vi "LCA Get Axis Handle.vi"(8 "error in (no error)":errorcluster caption="Fehler (Eingang, kein Fehler)", 10 "Axis Index":u8, 11 "Axis System Handle":i64) -> (0 "error out":errorcluster caption="Fehler (Ausgang)", 3 "AxisHandle":i64)   [LabVIEW 2021, in "labbCAN_MotionControl_API.lvlib"]
doc: "LCA_Func dev_hdl __stdcall LCA_GetAxisHandle(dev_hdl hAxisSystem,\n unsigned char AxisId);"
uses:
  labbCAN_MotionControl_API.lvlib
  labbCAN_MotionControl_API.dll
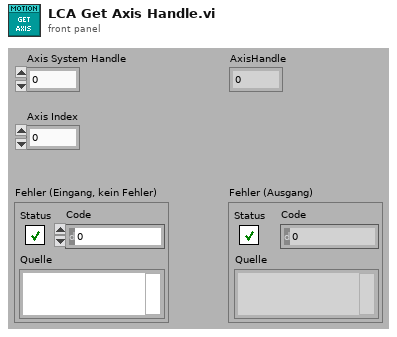
[diagram p1: front panel]
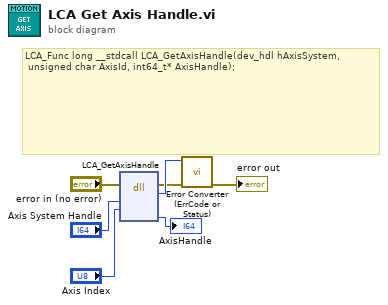
[diagram p0: block diagram]
diagram:
  # "LCA_Func long __stdcall LCA_GetAxisHandle(dev_hdl hAxisSystem,\n\tunsigned char AxisId, int64_t* AxisHandle);"
  n1 = dll-call lib="C:/Users/olaja/AppData/Local/CETONI_SDK/labbCAN_MotionControl_API.*" fn="LCA_GetAxisHandle"(error in="error in (no error)", "hAxisSystem"="Axis System Handle", "AxisId"="Axis Index") -> (error out=w3:errorcluster, "Rückgabetyp"=w7:i32, "AxisHandle"=→"AxisHandle":i64)  [unwired: 5 in, 1 out]
  n2 = call "Error Converter (ErrCode or Status).vi"("error in (no error)"=w3, "error code"=w7) -> ("error out"=→"error out":errorcluster)  [unwired: 9 in]
